vi "Read Accounts Files.vi"(8 "error in (no error)":errorcluster, 11 "Module Data":T1={"UI Controls"={"ATM Messages"=refnum, "User Input"=refnum, "Right Buttons"=refnum, "Right Menu"=refnum, "Left Buttons"=refnum, "Left Menu"=refnum, "Card Simulator"=refnum, "Enter"=refnum}, "ATM Messages 2"={"Session terminate message"="Your session has been terminated\ndue to inactivity or menu selection.\nPlease take your card\n\nGoodbye!", "Welcome message"="Welcome to Acme bank.\nPlease insert your card\nand enter your account\nnumber in the User Input.\n\nPress Enter (E) when done.", "Deposit Message"="Please enter amount to deposit and press\nEnter (E) when done.", "Deposit Complete Message"="$ (Amount) Deposited", "Withdrawal Message"="Please enter amount to withdraw and press\nEnter (E) when done.", "Withdrawal Complete Message"="$ (Amount) Withdrawn", "Balance Inquiry Message"="Your Balance Is:\n$ (Balance amount from file)", "Account verification failed message"="Account information incorrect\nPlease Re-Enter Account Number.\nPress Enter (E) when done.", "Withdrawal failed message"="Insufficient funds in account\nplease check your balance\nand try again", "Card Inserted"="Card Inserted", "Main Menu message"="Welcome to Acme bank.\nFirst name, last Name (from file)\n\nplease select transaction\nby using the buttons."}, "User Input"="", "ATM Messages"="", "Acc. file path"=path "", "Accounts Data"=[], "User Input Data"={"Account No"="", "Amount"="", "Activity"=enum."Fast Cash $50"}, "Message"=""}) -> (0 "error out":errorcluster, 1 "all rows":string[][](array[string]), 2 "Balances Column":string[](array[string]), 3 "Acc Numbers Column":string[](array[string]))   [LabVIEW 2016]
doc: "Read account.txt and index account number column and balance column.s"
uses:
  <vilib>/Utility/file.llb/Read Delimited Spreadsheet (string).vi
  Controls/UI Controls.ctl
  Controls/ATM Messages.ctl
  Controls/Module Data.ctl
  Controls/User Input Data.ctl
  Controls/Transaction Status.ctl
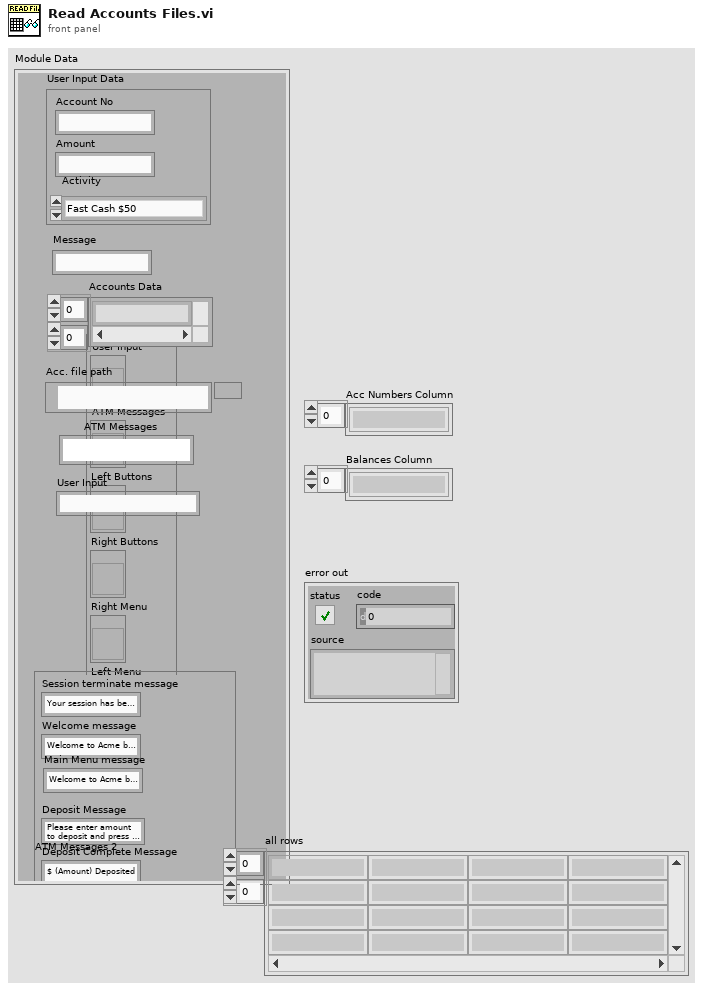
[diagram p1: front panel]
types:
  T1 = typedef "Module Data.ctl" = cluster{"UI Controls":T2, "ATM Messages 2":T3, "User Input":string, "ATM Messages":string, "Acc. file path":path, "Accounts Data":string[][], "User Input Data":T4, "Message":string}
  T2 = typedef "UI Controls.ctl" = cluster{"ATM Messages":refnum<vi>, "User Input":refnum<vi>, "Right Buttons":refnum<vi>, "Right Menu":refnum<vi>, "Left Buttons":refnum<vi>, "Left Menu":refnum<vi>, "Card Simulator":refnum<vi>, "Enter":refnum<vi>}
  T3 = typedef "ATM Messages.ctl" = cluster{"Session terminate message":string, "Welcome message":string, "Deposit Message":string, "Deposit Complete Message":string, "Withdrawal Message":string, "Withdrawal Complete Message":string, "Balance Inquiry Message":string, "Account verification failed message":string, "Withdrawal failed message":string, "Card Inserted":string, "Main Menu message":string}
  T4 = typedef "User Input Data.ctl" = cluster{"Account No":string, "Amount":string, "Activity":T5}
  T5 = typedef "Transaction Status.ctl" = enum16{"Fast Cash $50", "Withdrawal?", "Deposit?", "Account Number?"}
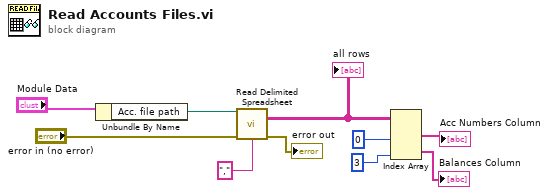
[diagram p0: block diagram]
diagram:
  n1 = Unbundle By Name("Module Data") -> ("Acc. file path"=w6:path)
  n2 = call-poly <vilib>:"Read Delimited Spreadsheet.vi"("file path (dialog if empty)"=w6, "error in (no error)"="error in (no error)", "delimiter (\\t)"="," ("delimiter (\\t)")) -> ("all rows"=w2:string[][], "error out"=→"error out":errorcluster)  [unwired: 7 in, 4 out]
  "all rows" <- w2
  n3 = Index Array(array=w2, index (col) #1=0 ("disabled index (col)"), index (col) #2=3 ("index (col)")) -> (element #1=→"Acc Numbers Column":string[], element #2=→"Balances Column":string[])  [unwired: 2 in]
